vi "WPS_control.vi"(0 "Path to Batch":string, 1 "Path to Exe":string, 2 "WPS IP:Port":string, 3 "Username":string, 4 "Password":string, 5 "Outlet Array":T1(array[cluster])) -> (14 "Standard Output":string[](array[string]), 19 "error out":errorcluster)   [LabVIEW 2009]
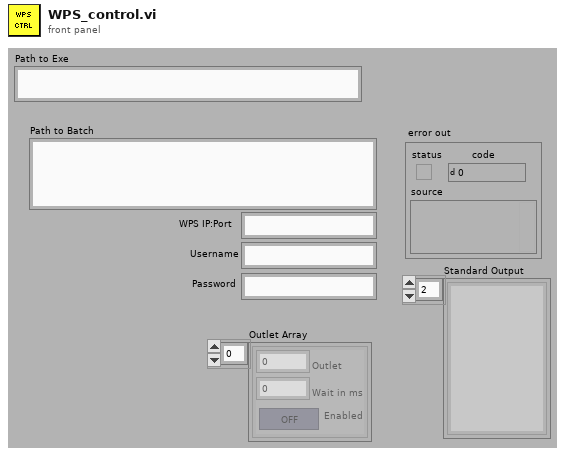
[diagram p1: front panel]
types:
  T1 = cluster{"Outlet":u32, "Wait in ms":u32, "Enabled":bool}[]
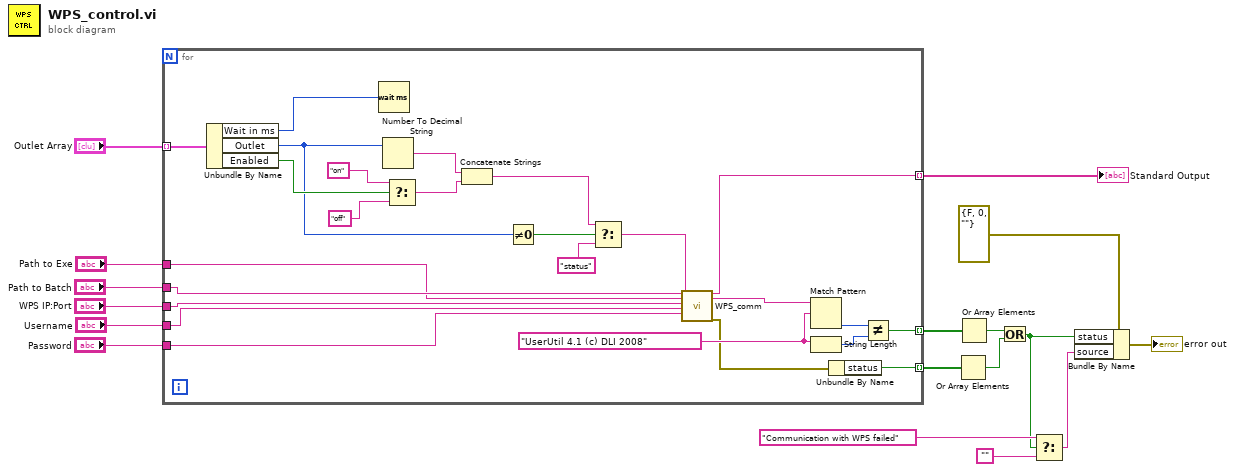
[diagram p0: block diagram]
diagram:
  n1 = for {
    tunnel: "Outlet Array" -> [w42] mode=indexing
    tunnel: "Path to Batch" -> [w36]
    tunnel: "Username" -> [w35]
    tunnel: "WPS IP:Port" -> [w34]
    tunnel: "Password" -> [w33]
    tunnel: [w28] -> w12 mode=indexing
    tunnel: [w26] -> w11 mode=indexing
    tunnel: [w24] -> w2 mode=indexing
    tunnel: "Path to Exe" -> [w18]
    w31 = "UserUtil 4.1 (c) DLI 2008"
    n2 = Unbundle By Name(w42) -> ("Wait in ms"=w41:u32, "Outlet"=w23:u32, "Enabled"=w25:bool)
    n3 = Wait (ms)(milliseconds to wait=w41) -> ()  [unwired: 1 out]
    n4 = Number To Decimal String(number=w23) -> (decimal integer string=w38:string)  [unwired: 1 in]
    n5 = Select(t="on", s=w25, f="off") -> (s? t:f=w37:string)
    n6 = Concatenate Strings(w38, w37) -> (w21:string)
    n7 = Not Equal To 0?(x=w23) -> (x != 0?=w22:bool)
    n8 = Select(t=w21, s=w22, f="status") -> (s? t:f=w19:string)
    n9 = call "WPS_comm.vi"("Path to Batch"=w36, "Path to Exe"=w18, "WPS IP:Port"=w34, "Username"=w35, "Password"=w33, "Command"=w19) -> ("standard output"=w24:string, "standard error"=w32:string, "error out"=w27:errorcluster)  [unwired: 10 in, 1 out]
    n10 = Match Pattern(string=w32, regular expression=w31) -> (offset past match=w30:i32)  [unwired: 1 in, 3 out]
    n11 = String Length(string=w31) -> (length=w29:i32)
    n12 = Unbundle By Name(w27) -> ("status"=w26:bool)
    n13 = Not Equal?(x=w30, y=w29) -> (x != y?=w28:bool)
  }
  "Standard Output" <- w2
  n14 = Or Array Elements(Boolean array=w11) -> (logical OR=w9:bool)
  n15 = Or Array Elements(Boolean array=w12) -> (logical OR=w10:bool)
  n16 = Or(x=w10, y=w9) -> (x .or. y?=w6:bool)
  n17 = Select(t="Communication with WPS failed", s=w6, f="") -> (s? t:f=w5:string)
  n18 = Bundle By Name(cluster=errorcluster {"status"=FALSE, "code"=0, "source"=""} ("error out"), "status"=w6, "source"=w5) -> (→"error out":errorcluster)
